vi "adlink7230ReadAndWriteIO.vi"(6 "Digital Output":bool[](array[boolean])=[TRUE, TRUE, TRUE, TRUE, TRUE, TRUE, TRUE, TRUE], 8 "error in (no error)":errorcluster caption="错误输入（无错误）", 9 "输出OUTPUT 2":T1, 10 "task in Output":refnum<k7>, 11 "task in Input":refnum<k7>) -> (0 "error out":errorcluster caption="错误输出", 1 "输入INPUT 2":T2, 2 "task out Output":refnum<k7>, 3 "task out Input":refnum<k7>, 4 "Digital Input":bool[](array[boolean]))   [LabVIEW 2017]
uses:
  <userlib>/DAQPilot/write.llb/PLT Write (Digital 1D Bool 1Chan 1Samp).vi
  <userlib>/DAQPilot/read.llb/PLT Read (Digital 1D Bool 1Chan 1Samp).vi
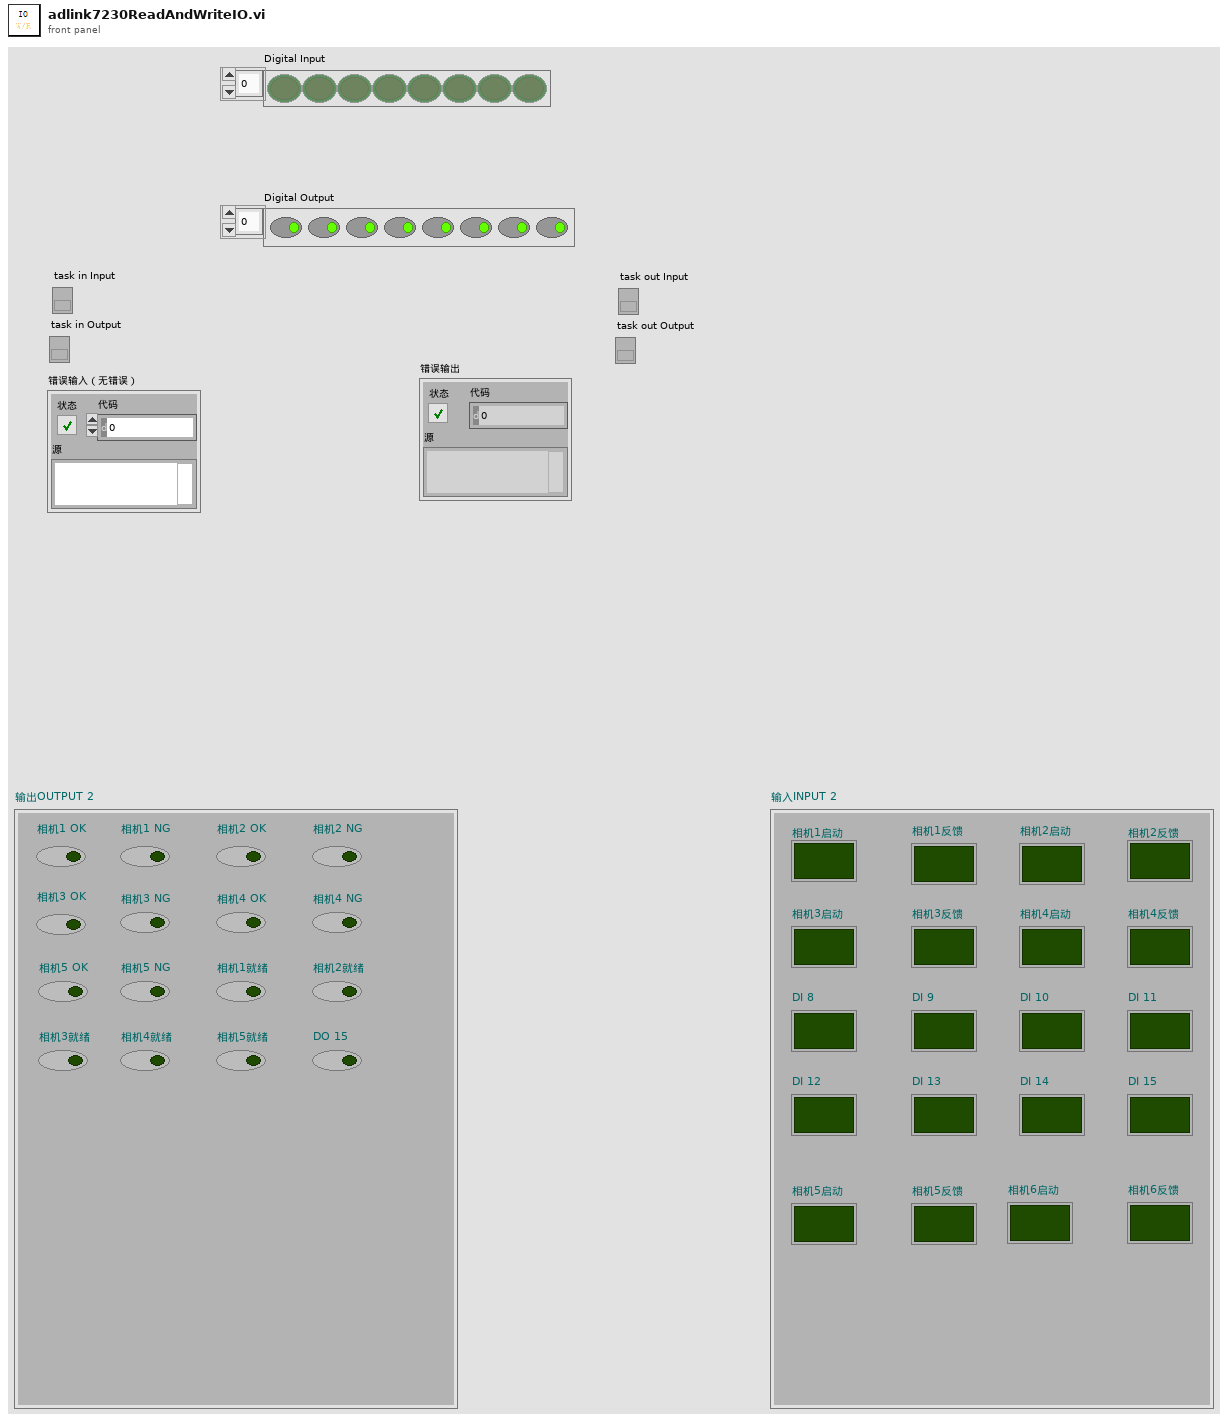
[diagram p1: front panel]
types:
  T1 = cluster{"相机1 OK":bool, "相机1 NG":bool, "相机2 OK":bool, "相机2 NG":bool, "相机3 OK":bool, "相机3 NG":bool, "相机4 OK":bool, "相机4 NG":bool, "相机5 OK":bool, "相机5 NG":bool, "相机1就绪":bool, "相机2就绪":bool, "相机3就绪":bool, "相机4就绪":bool, "相机5就绪":bool, "DO 15":bool}
  T2 = cluster{"相机1启动":bool, "相机1反馈":bool, "相机2启动":bool, "相机2反馈":bool, "相机3启动":bool, "相机3反馈":bool, "相机4启动":bool, "相机4反馈":bool, "DI 8":bool, "DI 9":bool, "DI 10":bool, "DI 11":bool, "DI 12":bool, "DI 13":bool, "DI 14":bool, "DI 15":bool, "相机5启动":bool, "相机5反馈":bool, "相机6启动":bool, "相机6反馈":bool}
  T3 = cluster{"相机1启动":bool, "相机1反馈":bool, "相机2启动":bool, "相机2反馈":bool, "相机3启动":bool, "相机3反馈":bool, "相机4启动":bool, "相机4反馈":bool, "DI 8":bool, "DI 9":bool, "DI 10":bool, "DI 11":bool, "DI 12":bool, "DI 13":bool, "DI 14":bool, "DI 15":bool}
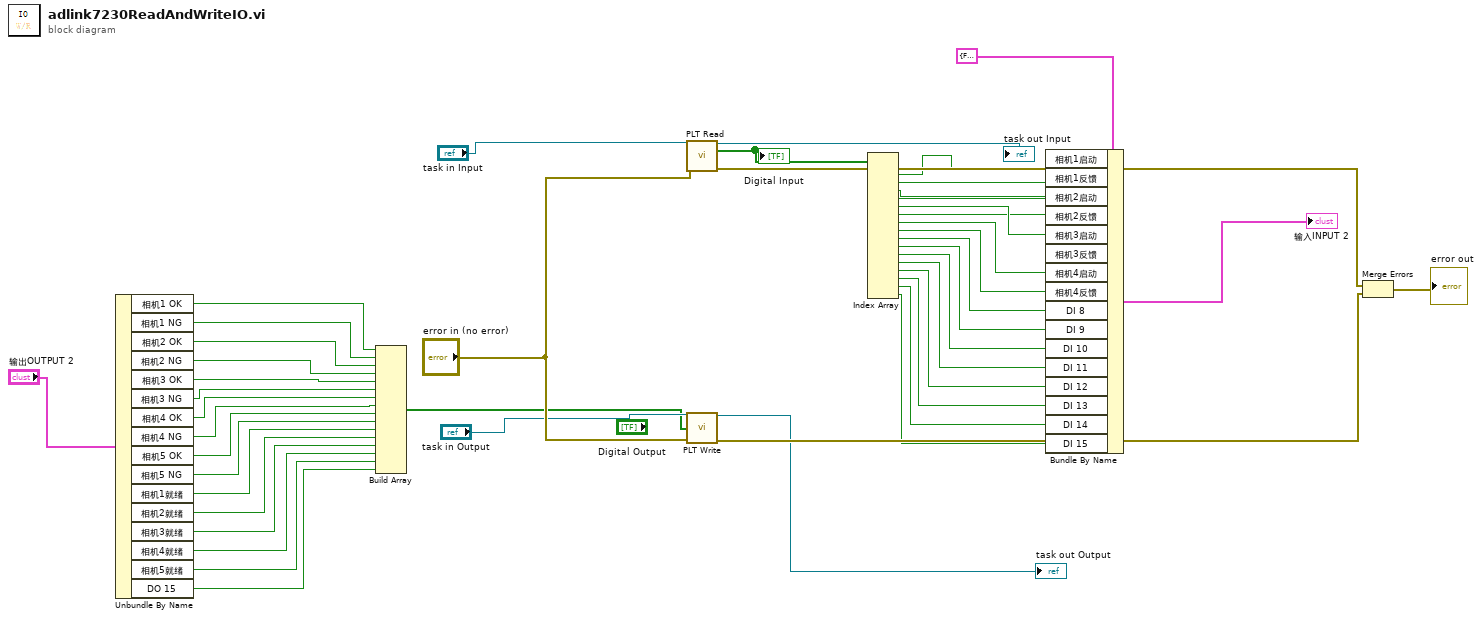
[diagram p0: block diagram]
diagram:
  n1 = Unbundle By Name("输出OUTPUT 2") -> ("相机1 OK"=w28:bool, "相机1 NG"=w27:bool, "相机2 OK"=w26:bool, "相机2 NG"=w25:bool, "相机3 OK"=w24:bool, "相机3 NG"=w23:bool, "相机4 OK"=w22:bool, "相机4 NG"=w21:bool, "相机5 OK"=w16:bool, "相机5 NG"=w15:bool, "相机1就绪"=w14:bool, "相机2就绪"=w13:bool, "相机3就绪"=w12:bool, "相机4就绪"=w11:bool, "相机5就绪"=w10:bool, "DO 15"=w9:bool)
  n2 = Build Array(w28, w27, w26, w25, w24, w23, w22, w21, w16, w15, w14, w13, w12, w11, w10, w9) -> (w20:bool[])
  n3 = call-poly <userlib>:"PLT Read.vi"("task/channels in"="task in Input", "error in"="error in (no error)") -> ("task out"=→"task out Input":refnum<k7>, "data"=w37:bool[], "error out"=w42:errorcluster)  [unwired: 11 in]
  "Digital Input" <- w37
  n4 = call-poly <userlib>:"PLT Write.vi"("task/channels in"="task in Output", "data"=w20, "error in"="error in (no error)") -> ("task out"=→"task out Output":refnum<k7>, "error out"=w41:errorcluster)  [unwired: 10 in, 1 out]
  n5 = Index Array(array=w37) -> (element #1=w36:bool, element #2=w35:bool, element #3=w34:bool, element #4=w33:bool, element #5=w32:bool, element #6=w31:bool, element #7=w30:bool, element #8=w29:bool, element #9=w8:bool, element #10=w7:bool, element #11=w6:bool, element #12=w5:bool, element #13=w4:bool, element #14=w3:bool, element #15=w2:bool, element #16=w1:bool)  [unwired: 16 in]
  n6 = Bundle By Name(cluster=T3 {"相机1启动"=FALSE, "相机1反馈"=FALSE, "相机2启动"=FALSE, "相机2反馈"=FALSE, "相机3启动"=FALSE, "相机3反馈"=FALSE, "相机4启动"=FALSE, "相机4反馈"=FALSE, "DI 8"=FALSE, "DI 9"=FALSE, "DI 10"=FALSE, "DI 11"=FALSE, "DI 12"=FALSE, "DI 13"=FALSE, "DI 14"=FALSE, "DI 15"=FALSE} ("输入INPUT 2"), "相机1启动"=w36, "相机1反馈"=w35, "相机2启动"=w34, "相机2反馈"=w33, "相机3启动"=w32, "相机3反馈"=w31, "相机4启动"=w30, "相机4反馈"=w29, "DI 8"=w8, "DI 9"=w7, "DI 10"=w6, "DI 11"=w5, "DI 12"=w4, "DI 13"=w3, "DI 14"=w2, "DI 15"=w1) -> (→"输入INPUT 2":T3)
  n7 = Merge Errors(w42, w41) -> (→"error out":errorcluster)
